vi "check_error.vi"(8 "error in":errorcluster) -> (0 "error out":errorcluster)   [LabVIEW 2011, in "Fiberscope_library.lvlib"]
uses:
  Fiberscope_library.lvlib
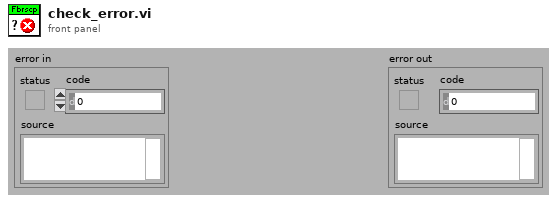
[diagram p1: front panel]
types:
  T1 = cluster{"error in (no error)":errorcluster, string}
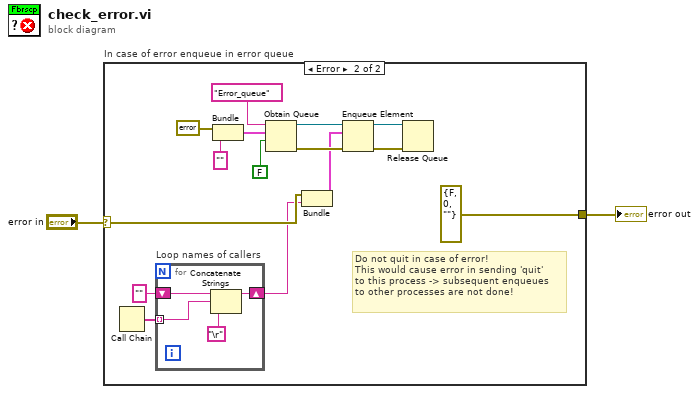
[diagram p0: block diagram]
diagram:
  n1 = case "In case of error enqueue in error queue" shown="Error" "error in" {
    selector: "error in" -> [w3 w8]
    tunnel: [w3 errorcluster {"status"=FALSE, "code"=0, "source"=""} ("error IO")] -> w1
    frame No Error {
    }
    frame Error {
      # "Do not quit in case of error!\nThis would cause error in sending 'quit'\nto this process -> subsequent enqueues\nto other processes are not done!"
      n2 = Call Chain() -> (call chain=w9:string[])
      n3 = for "Loop names of callers" {
        tunnel: w9 -> [w22] mode=indexing
        shift-right: [w21] -> w4
        shift-left: "" -> [w20]
        n4 = Concatenate Strings(w20, w22, "\r") -> (w21:string)
      }
      n5 = Bundle("error in (no error)"=errorcluster {"status"=FALSE, "code"=0, "source"=""}, "") -> (w10:T1)  [unwired: 1 in]
      n6 = Obtain Queue(name (unnamed)="Error_queue", element data type=w10, create if not found? (T)=FALSE) -> (queue out=w17:refnum<queue>, error out=w15:errorcluster)  [unwired: 2 in, 1 out]
      n7 = Bundle("error IO"=w8, w4) -> (w7:cluster{"error IO":errorcluster, string})  [unwired: 1 in]
      n8 = Enqueue Element(queue=w17, element=w7, error in (no error)=w15) -> (queue out=w16:refnum<queue>, error out=w14:errorcluster)  [unwired: 1 in, 1 out]
      n9 = Release Queue(queue=w16, error in (no error)=w14) -> ()  [unwired: 1 in, 3 out]
    }
  }
  "error out" <- w1
